vi "Connect.vi"(0 "OWEN HMI in":refnum<class "OWEN HMI.lvclass">, 11 "error in (no error)":errorcluster) -> (4 "OWEN HMI out":refnum<class "OWEN HMI.lvclass">, 15 "error out":errorcluster)   [LabVIEW 2019, in "OWEN HMI.lvclass"]
uses:
  OWEN HMI.lvclass
  OWEN HMI.lvclass/OWEN HMI.ctl
  <vilib>/NI/Modbus Library/API/Wrapper/Create TCP Master.vi
  <vilib>/NI/Modbus Library/API/Master/Modbus Master.lvclass
  <vilib>/NI/Modbus Library/API/Wrapper/API Main.lvlib
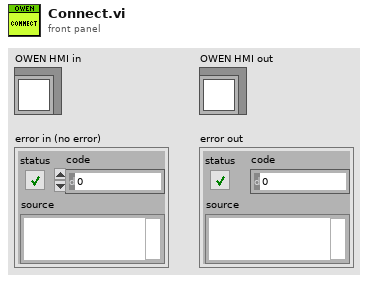
[diagram p1: front panel]
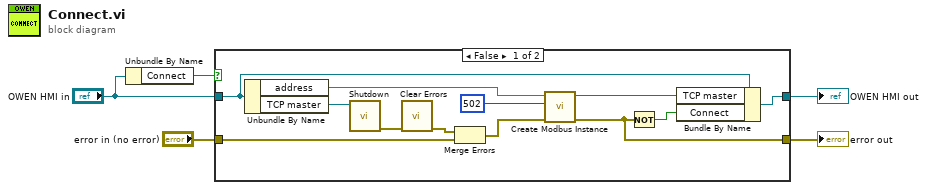
[diagram p0: block diagram]
diagram:
  n1 = Unbundle By Name("OWEN HMI in") -> ("Connect"=w5:bool)
  n2 = case shown="False" w5 {
    tunnel: "OWEN HMI in" -> [w11 w19]
    tunnel: [w15 w18] -> w2
    tunnel: [w13 w19] -> w3
    tunnel: "error in (no error)" -> [w12 w18]
    frame False {
      n3 = Unbundle By Name(w11) -> ("address"=w10:string, "TCP master"=w9:refnum<class "Modbus Master.lvclass">)
      n4 = call-dynamic "Shutdown.vi"("Modbus master in"=w9) -> ("error out"=w8:errorcluster)  [unwired: 10 in]
      n5 = call <vilib>:"Clear Errors.vi"("error in (no error)"=w8) -> ("error out"=w6:errorcluster)  [unwired: 5 in, 1 out]
      n6 = Merge Errors(w6, w12) -> (w7:errorcluster)
      n7 = call-poly <vilib>:"Create Modbus Instance.vi"("error in"=w7, "port (502)"=u16 502, "address"=w10) -> ("error out"=w15:errorcluster, "TCP master instance"=w16:refnum<class "Modbus Master.lvclass">)  [unwired: 7 in]
      n8 = Not(x=w15) -> (.not. x?=w14:bool)
      n9 = Bundle By Name(cluster=w11, "TCP master"=w16, "Connect"=w14) -> (w13:refnum<class "OWEN HMI.lvclass">)
    }
    frame True {
    }
  }
  "OWEN HMI out" <- w3
  "error out" <- w2
